vi "Get All Users Directory.vi"() -> (0 "All User Path":path)   [LabVIEW 2016]
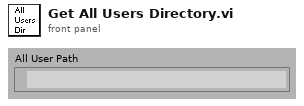
[diagram p1: front panel]
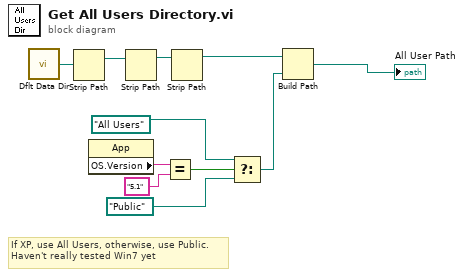
[diagram p0: block diagram]
diagram:
  # "If XP, use All Users, otherwise, use Public.\nHaven't really tested Win7 yet"
  n1 = call <vilib>:"Dflt Data Dir.vi"() -> ("App:Default Data Directory"=w5:path)
  n2 = Strip Path(path=w5) -> (stripped path=w6:path)  [unwired: 1 out]
  n3 = property class="App"() -> ("OS.Version"=w7:string)  [unwired: 2 in, 2 out]
  n4 = Strip Path(path=w6) -> (stripped path=w4:path)  [unwired: 1 out]
  n5 = Equal?(x=w7, y="5.1") -> (x = y?=w9:bool)
  n6 = Strip Path(path=w4) -> (stripped path=w3:path)  [unwired: 1 out]
  n7 = Select(t=path "All Users", s=w9, f=path "Public") -> (s? t:f=w2:path)
  n8 = Build Path(base path=w3, name or relative path=w2) -> (appended path=→"All User Path":path)
